vi "readTriggerCoupling.vi"(8 "error in (no error)":errorcluster, 9 "Coupling":T1, 10 "output cluster out":T2, 11 "IVI Refnum in":refnum<k15>) -> (0 "error out":errorcluster, 2 "output cluster":T2={"DC Restore"=enum."off", "Polarity"=enum."Negative", "TV Event"=enum."Field 1", "Coupling"=enum."AC", "Slope"=enum."Negative", "AnalogSource"=enum."Channel 0", "Window Mode"=enum."Entering", "Low Level"=0.0, "High Level"=0.0, "Hysteresis"=0.0, "Delay"=0.0, "Holdoff"=0.0, "Signal Format"=enum."M-NTSC", "Mode"=enum."Immediate", "Line Number"=0, "DigitalSource"=enum."RTSI 0"}, 3 "IVI Refnum out":refnum<k15>)   [LabVIEW 2011]
uses:
  TriggerSettings_TypDef.ctl
  OnOffTypeDef.ctl
  Polarity_TypDEf.ctl
  TVEvent_TypDef.ctl
  coupling_TypDef.ctl
  positive_negatice2_typDef.ctl
  TriggerSource_TypDef.ctl
  triggerwindowmode2_TypDef.ctl
  SignalFormat_TypDef.ctl
  mode_TypDef.ctl
  Trigger.DigitalSource_TypDEf.ctl
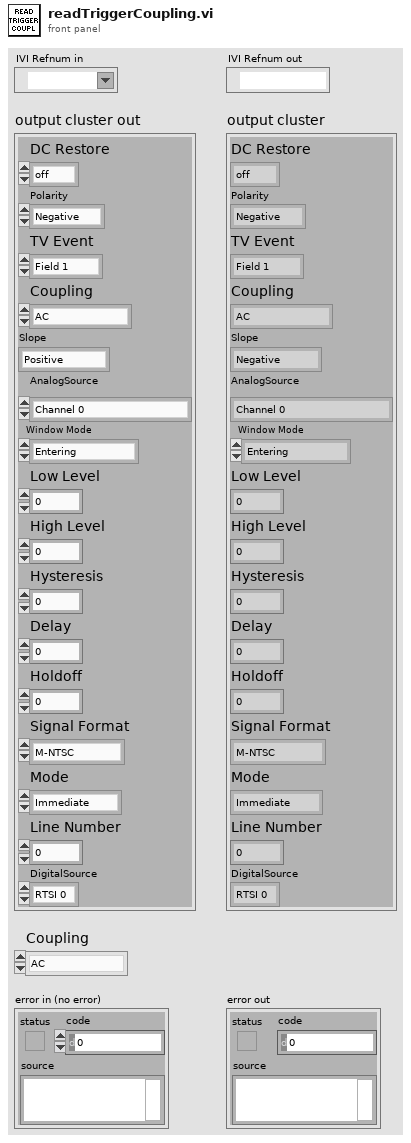
[diagram p1: front panel]
types:
  T1 = typedef "coupling_TypDef.ctl" = enum16{"AC", "DC", "HF Reject", "LF Reject", "AC Plus HF Reject"}
  T2 = typedef "TriggerSettings_TypDef.ctl" = cluster{"DC Restore":T3, "Polarity":T4, "TV Event":T5, "Coupling":T1, "Slope":T6, "AnalogSource":T7, "Window Mode":T8, "Low Level":dbl, "High Level":dbl, "Hysteresis":dbl, "Delay":dbl, "Holdoff":dbl, "Signal Format":T9, "Mode":T10, "Line Number":i32, "DigitalSource":T11}
  T3 = typedef "OnOffTypeDef.ctl" = enum16{"off", "on"}
  T4 = typedef "Polarity_TypDEf.ctl" = enum16{"Negative", "Positive"}
  T5 = typedef "TVEvent_TypDef.ctl" = enum16{"Field 1", "Field 2", "Any Field", "Any Line", "Line Number"}
  T6 = typedef "positive_negatice2_typDef.ctl" = enum16{"Positive", "Negative"}
  T7 = typedef "TriggerSource_TypDef.ctl" = enum16{"Channel 0", "Channel 1", "External TRIG"}
  T8 = typedef "triggerwindowmode2_TypDef.ctl" = enum16{"Entering", "Leaving"}
  T9 = typedef "SignalFormat_TypDef.ctl" = enum16{"M-NTSC", "B/G-PAL", "SECAM", "M-PAL", "480i/59.94 fps", "480i/60 fps", "480p/59.94 Fps", "480p/60 Fps", "576i/50 fps", "576p/50 Fps", "720p/50 Fps", "720p/59.94 Fps", "720p/60 Fps", "1080i/50 fps", "1080i/59.94 fps", "1080i/60 fps", "1080p/24 Fps"}
  T10 = typedef "mode_TypDef.ctl" = enum32{"Immediate", "Analog Edge", "Analog Window", "Analog Hysteresis", "Video", "Digital Edge"}
  T11 = typedef "Trigger.DigitalSource_TypDEf.ctl" = enum16{"RTSI 0", "RTSI 1", "RTSI 2", "RTSI 3", "RTSI 4", "RTSI 5", "RTSI 6", "PFI 0", "PFI 1", "PFI 2", "PXI Star Trigger"}
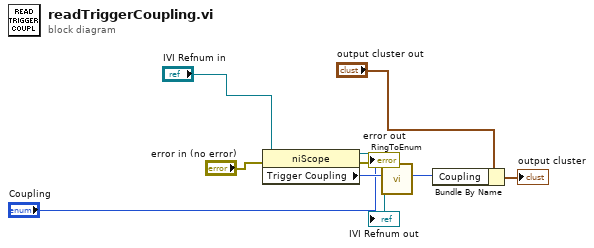
[diagram p0: block diagram]
diagram:
  n1 = property class="niScope"(reference="IVI Refnum in", error in="error in (no error)") -> (reference out=→"IVI Refnum out":refnum<k15>, error out=→"error out":errorcluster, "Trigger Coupling"=w3:i32)
  n2 = call "RingToEnum.vi"("Numeric"=w3, "Enum"="Coupling") -> ("Value"=w5:i32)  [unwired: 9 in]
  n3 = Bundle By Name(cluster="output cluster out", "Coupling"=w5) -> (→"output cluster":T2)
